vi "amplitude_sweep_stimulus.vi"(1 "Parameters":T1={"Length (sec)"=5.0, "Initial amplitude"=0.15, "Frequency (Hz)"=1.0, "Nonlinearity"=150.0} {"Nonlinearity" format="%#_3p"; "Frequency (Hz)" format="%#_3p"; "Initial amplitude" format="%#_3p"; "Length (sec)" format="%#_3p"}) -> (0 "Result":sgl[][](array[numeric]))   [LabVIEW 2013]
panel:
  out "Waveform Graph":sgl[](graph)
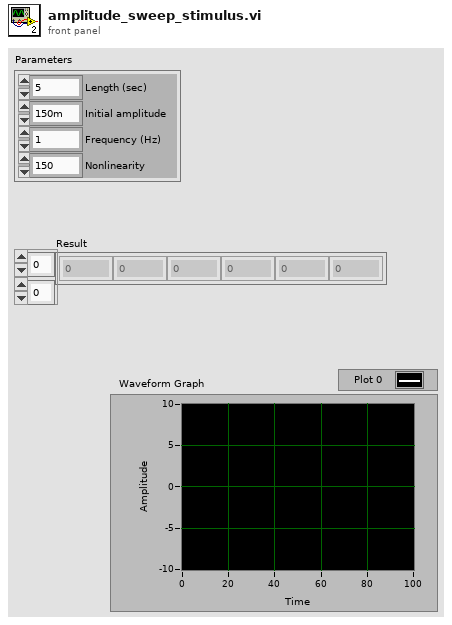
[diagram p1: front panel]
types:
  T1 = cluster{"Length (sec)":sgl, "Initial amplitude":sgl, "Frequency (Hz)":sgl, "Nonlinearity":sgl}
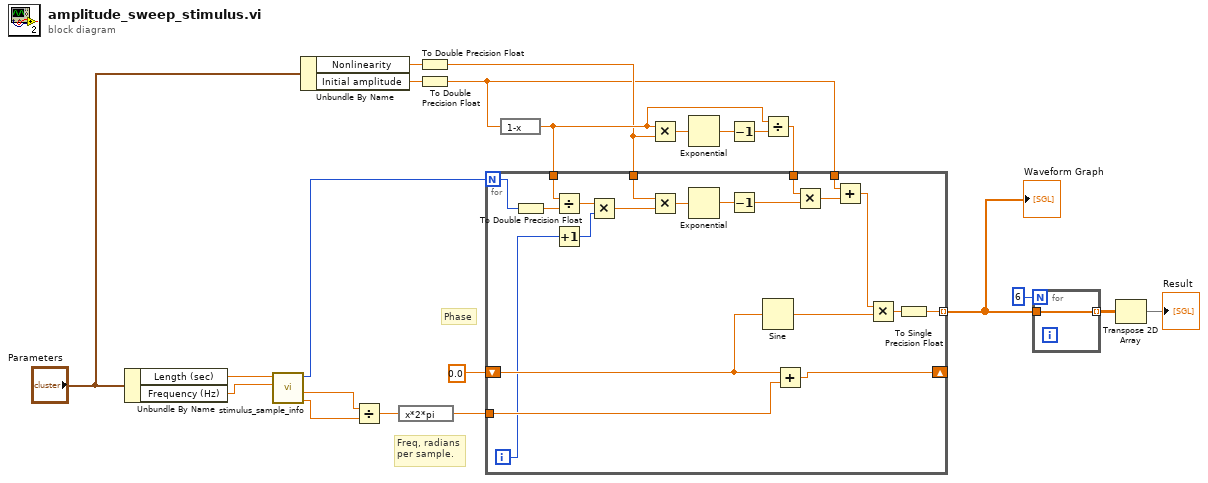
[diagram p0: block diagram]
diagram:
  # "Freq, radians\nper sample."
  # "Phase"
  n1 = Unbundle By Name("Parameters") -> ("Length (sec)"=w10:sgl, "Frequency (Hz)"=w9:sgl)
  n2 = call "stimulus_sample_info.vi"("Frequency"=w9, "Length"=w10) -> ("Sample frequency"=w6:dbl, "Actual frequency"=w7:dbl, "Num samples"=w22:i32)  [unwired: 6 in, 1 out]
  n3 = Unbundle By Name("Parameters") -> ("Nonlinearity"=w5:sgl, "Initial amplitude"=w3:sgl)
  n4 = Divide(x=w7, y=w6) -> (x/y=w17:dbl)
  n5 = expression code="x*2*pi"(w17) -> (w16:dbl)
  n6 = To Double Precision Float(number=w5) -> (double precision float=w4:dbl)
  n7 = To Double Precision Float(number=w3) -> (double precision float=w2:dbl)
  n8 = expression code="1-x"(w2) -> (w11:dbl)
  n9 = Multiply(x=w11, y=w4) -> (x*y=w12:dbl)
  n10 = Exponential(1:w12) -> (0:w13:dbl)
  n11 = Decrement(x=w13) -> (x-1=w14:dbl)
  n12 = Divide(x=w11, y=w14) -> (x/y=w15:dbl)
  n13 = for {
    N: w22 -> [w40]
    shift-right: [w43] -> _
    shift-left: 0.0 ("ln(x)") -> [w42]
    tunnel: [w23] -> w1 mode=indexing
    tunnel: w16 -> [w41]
    tunnel: w4 -> [w34]
    tunnel: w15 -> [w32]
    tunnel: w2 -> [w29]
    tunnel: w11 -> [w28]
    i -> [w36]
    n14 = To Double Precision Float(number=w40) -> (double precision float=w39:dbl)
    n15 = Divide(x=w28, y=w39) -> (x/y=w38:dbl)
    n16 = Increment(x=w36) -> (x+1=w37:i32)
    n17 = Multiply(x=w38, y=w37) -> (x*y=w35:dbl)
    n18 = Multiply(x=w34, y=w35) -> (x*y=w33:dbl)
    n19 = Exponential(1:w33) -> (0:w27:dbl)
    n20 = Decrement(x=w27) -> (x-1=w26:dbl)
    n21 = Sine(x=w42) -> (sin(x)=w25:dbl)
    n22 = Add(x=w42, y=w41) -> (x+y=w43:dbl)
    n23 = Multiply(x=w32, y=w26) -> (x*y=w31:dbl)
    n24 = Add(x=w29, y=w31) -> (x+y=w30:dbl)
    n25 = Multiply(x=w30, y=w25) -> (x*y=w24:dbl)
    n26 = To Single Precision Float(number=w24) -> (single precision float=w23:sgl)
  }
  "Waveform Graph" <- w1
  n27 = for {
    N: 6 -> [_]
    tunnel: w1 -> [w44]
    tunnel: [w44] -> w20 mode=indexing
  }
  n28 = Transpose 2D Array(2D array=w20) -> (transposed array=→"Result":sgl[][])
